vi "Teleop.vi"(10 "Match Info":T4={"Autonomous Elapsed Seconds"=0.0, "TeleOp Elapsed Seconds"=0.0, "Disabled Elapsed Seconds"=0.0, "Visited Autonomous"=FALSE, "Visited TeleOp"=FALSE, "Visited Disabled"=FALSE, "Autonomous Settings"={"Autonomous Style"=enum."Independent", "VI Refnum"=refnum}}, 11 "Call Context":T5) -> ()   [LabVIEW 2018]
doc: "This VI is called for each TeleOp packet received from the DS where the robot is not disabled. It is often used to read from the joysticks and update I/O or to update setpoints for timed control loops. It should complete and return within 20 milliseconds or it may miss DS packets."
uses:
  <vilib>/Rock Robotics/WPI/DriverStation/WPI_DriverStationDerivedRobotMode.ctl
  <vilib>/Rock Robotics/WPI/DriverStation/WPI_DriverStationMatch Info.ctl
  <vilib>/Rock Robotics/WPI/Solenoid/WPI_SolenoidValue.ctl
  <vilib>/Rock Robotics/WPI/ThirdParty/Phoenix-LabVIEW/Motor Controller/Controls/CTRE_Phoenix_MotorControl_ControlMode.ctl
  <vilib>/Rock Robotics/WPI/Switch/WPI_SwitchDevRef.ctl
  <vilib>/Rock Robotics/SystemInterfaces/DIO/FPGA_DIOChannel.ctl
  <vilib>/Rock Robotics/SystemInterfaces/Counter/FPGA_CounterCtrSystemIndex.ctl
  <vilib>/Rock Robotics/WPI/Utilities/WPI_GetSetVariantRefNum.vi
  <vilib>/Rock Robotics/WPI/Joystick/WPI_JoystickArcadeMapping.vi
  <vilib>/Rock Robotics/Network Tables/NT Write Boolean Array.vi
  <vilib>/Rock Robotics/Network Tables/NT Write Numeric Array.vi
  <vilib>/Rock Robotics/WPI/Solenoid/WPI_SolenoidSetEnum.vi
  <vilib>/Rock Robotics/WPI/ThirdParty/Phoenix-LabVIEW/Motor Controller/Get/CTRE_Phoenix_MotorController_GetSelectedSensorData.vi
  <vilib>/Rock Robotics/Network Tables/NT Read Boolean.vi
  Toolbox/Simple Limit Switch/Limits(Switch+Encoder).vi
  Toolbox/Simple Limit Switch/Limits(DoubleEncoder).vi
  Toolbox/Simple Limit Switch/Limits(DoubleSwitch).vi
  <vilib>/Rock Robotics/Network Tables/NT Read Number.vi
panel:
  in  "Reset Elevator Horse":bool
  out "OuterStageSwitch":bool
  out "Wrist Indicator":T1(ring)
  out "Elevator Intake":T2(ring)
  in  "Wrist":T1(ring)
  in  "Level":T2(ring)
  in  "Elevator Auto":bool
  in  "Elevator Output Range":cluster{"output high":dbl, "output low":dbl}={"output high"=0.25, "output low"=-0.25}
  in  "Elevator PID Gains":T3={"proportional gain (Kc)"=1.0, "integral time (Ti, min)"=0.01, "derivative time (Td, min)"=0.0}
  in  "Elevator Setpoints":dbl[](array[numeric])=[-1000.0, -100000.0, -250000.0, -250000.0, -270000.0, -480000.0]
  in  "Wrist Auto":bool
  in  "Wrist Output Range":cluster{"output high":dbl, "output low":dbl}={"output high"=0.25, "output low"=-0.25}
  in  "Wrist PID Gains":T3={"proportional gain (Kc)"=1.0, "integral time (Ti, min)"=0.01, "derivative time (Td, min)"=0.0}
  in  "Wrist Setpoints":dbl[](array[numeric])=[-34000.0, -34000.0, -34000.0, -34000.0, 120000.0, 50000.0, 38000.0, 0.0, -34000.0]
  in  "Level":i8
  in  "Into Home Limit Is Pos (Wrist)":bool
  out "Wrist Limit Switch":bool
  out "Elevator Limit Switch Top":bool
  in  "Into Home Limit Is Pos (Elevator)":bool=TRUE
  in  "Intake Encoder Limit":dbl=560000.0 format="%#_13g"
  in  "Intake Home Encoder Limit":dbl=-100000.0 format="%#_13g"
  in  "HorseDanger":i32=700
  in  "Horse Encoder Limit":dbl=180000.0 format="%#_13g"
  in  "Into Home Limit Is Pos (Horse)":bool
  out "Elevator Limit Switch":bool
  out "Elevator Encoder":i32
  in  "Reset Elevator Encoder":bool
  out "Horse Encoder":i32
  in  "Reset Wrist Encoder":bool
  out "Intake Wrist Encoder":i32
  # "UNKNOWN"
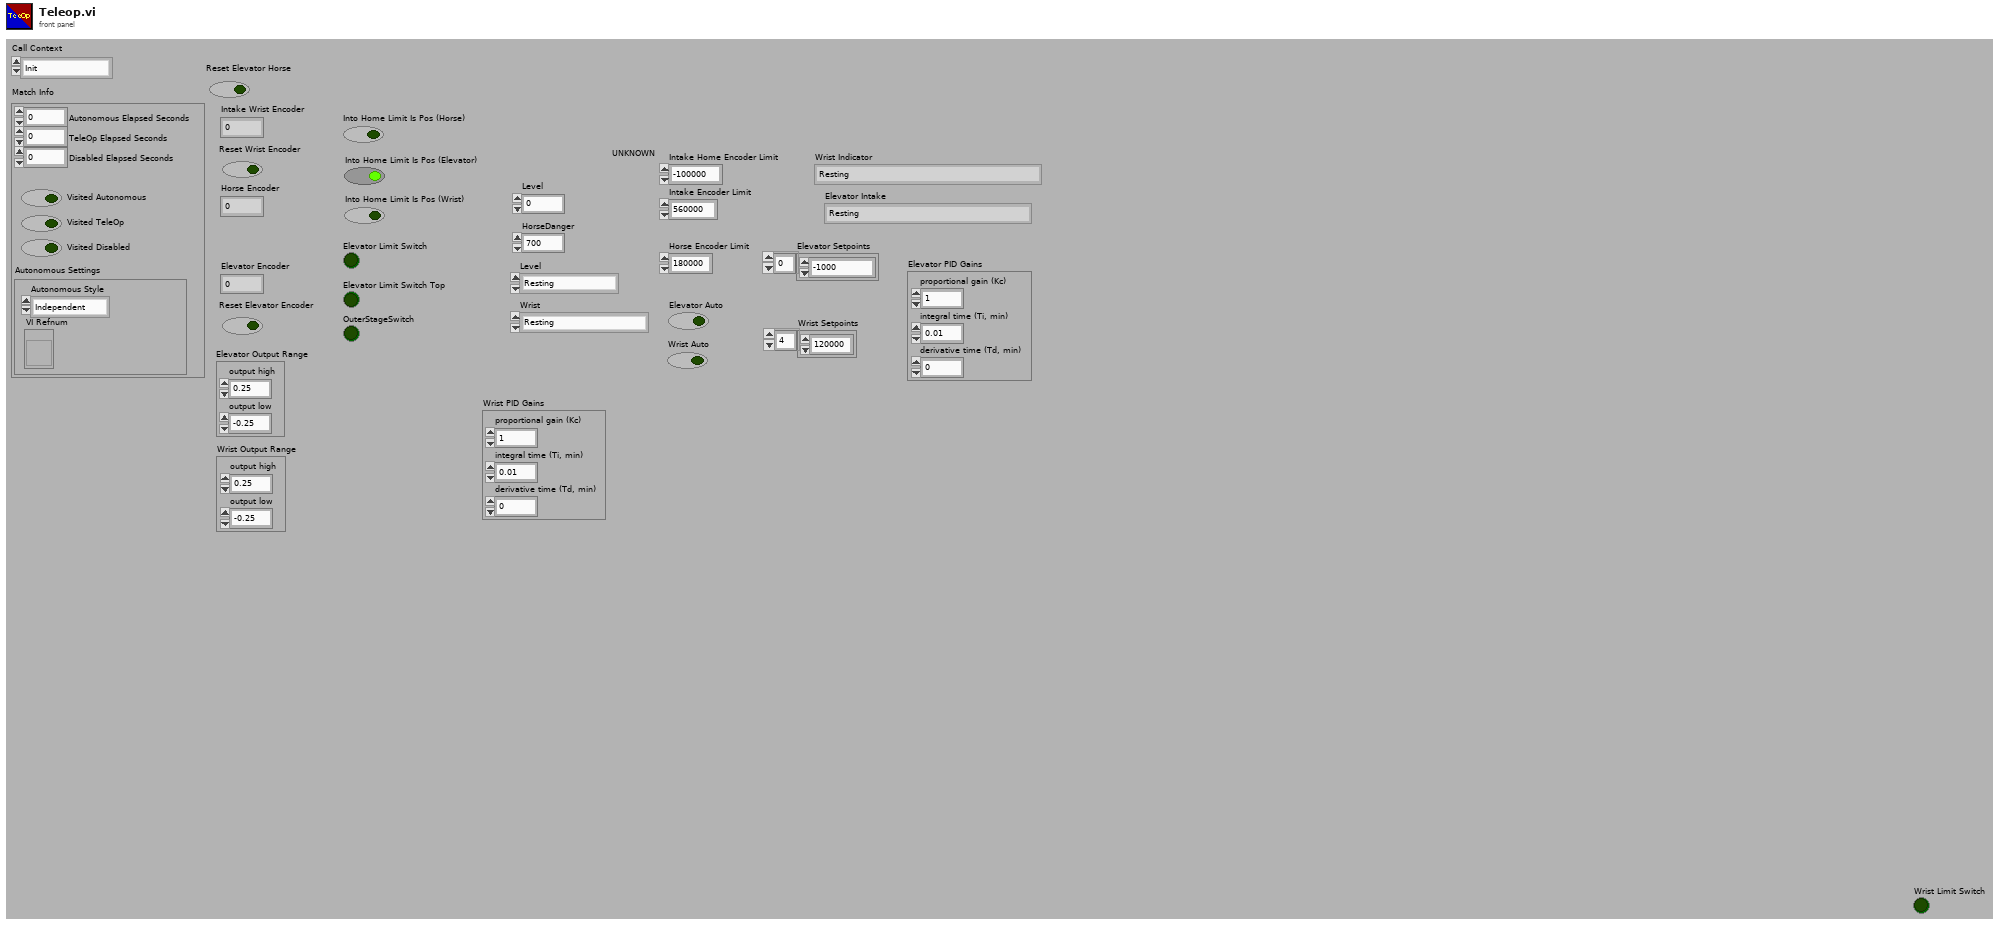
[diagram p1: front panel]
types:
  T1 = enum16{"Resting", "Hatch Ground Intake", "Hatch Place Low/Mid/CargoShip", "Hatch Place High", "Cargo Ground Intake", "Cargo Place Low/Mid", "Cargo Place High", "CargoShip Place Front", "CargoShip Place Back"}
  T2 = enum16{"Resting", "CargoShip Front", "CargoShip Back", "Cargo Mid", "Hatch Mid", "All High"}
  T3 = cluster{"proportional gain (Kc)":dbl, "integral time (Ti, min)":dbl, "derivative time (Td, min)":dbl}
  T4 = typedef "WPI_DriverStationMatch Info.ctl" = cluster{"Autonomous Elapsed Seconds":dbl, "TeleOp Elapsed Seconds":dbl, "Disabled Elapsed Seconds":dbl, "Visited Autonomous":bool, "Visited TeleOp":bool, "Visited Disabled":bool, "Autonomous Settings":cluster{"Autonomous Style":enum16{"Iterative", "Independent"}, "VI Refnum":refnum<vi>}}
  T5 = typedef "WPI_DriverStationDerivedRobotMode.ctl" = enum16{"Init", "Execute", "Stop"}
  T6 = typedef "WPI_SwitchDevRef.ctl" = cluster{"DevStatus":errorcluster, "DIO Channel":T7, "CntIndex":T8, "Normally Closed":bool}
  T7 = typedef "FPGA_DIOChannel.ctl" = enum8{"DIO 0", "DIO 1", "DIO 2", "DIO 3", "DIO 4", "DIO 5", "DIO 6", "DIO 7", "DIO 8", "DIO 9", "DIO MXP 0", "DIO MXP 1", "DIO MXP 2", "DIO MXP 3", "DIO MXP 4", "DIO MXP 5", "DIO MXP 6", "DIO MXP 7", "DIO MXP 8", "DIO MXP 9", "DIO MXP 10", "DIO MXP 11", "DIO MXP 12", "DIO MXP 13", "DIO MXP 14", "DIO MXP 15", "SPI Port CS1", "SPI Port CS2", "SPI Port CS3", "SPI Port MISO", "SPI Port MOSI", "Invalid"}
  T8 = typedef "FPGA_CounterCtrSystemIndex.ctl" = enum8{"Ctr 0", "Ctr 1", "Ctr 2", "Ctr 3", "Ctr 4", "Ctr 5", "Ctr 6", "Ctr 7", "Invalid"}
  T9 = cluster{"Increment Setpoint Index":bool, "Decrement Setpoint Index":bool}
  T10 = typedef "CTRE_Phoenix_MotorControl_ControlMode.ctl" = u16
  T11 = typedef "WPI_SolenoidValue.ctl" = enum16{"Off", "On", "Forward", "Reverse"}
  T12 = cluster{"Intake Wheels Forwards":bool, "Elevator Shift":bool, "Intake Wheels Backwards":bool, "Drivetrain Shift":bool, "Elevator Outer Forwards":bool, "Elevator Outer Backwards":bool, "Horse Drive Climber":bool, "Horse Drive Pistons":bool, "Horse Drive Up":bool, "Horse Drive Down":bool}
  T13 = typedef "WPI_JoystickDevRef.ctl" = cluster{"Device":T14}
  T14 = typedef "WPI_JoystickDeviceEnum.ctl" = enum16{"USB 0", "USB 1", "USB 2", "USB 3", "USB 4", "USB 5"}
  T15 = typedef "WPI_MotorControlDeviceRef.ctl" = cluster{"DeviceStatus":errorcluster, "Type":T16, "PWM":cluster{"PWM Channel":T17, "DeadBand":T18}, "CAN":cluster{"Device Number":u8, "SetOutput VI Ref":variant, "GetOutput VI Ref":variant, "Enable VI Ref":variant, "Disable VI Ref":variant, "Data":variant}, "Invert":bool, "DIO PWM":cluster{"PWM \"Enable\" Channel":T17, "DIOChannel":T7, "PWM Rate":dbl}}
  T16 = typedef "WPI_MotorControlType.ctl" = enum16{"PWM", "CAN", "DIO PWM"}
  T17 = typedef "FPGA_DIOPWMChannel.ctl" = enum8{"PWM 0", "PWM 1", "PWM 2", "PWM 3", "PWM 4", "PWM 5", "PWM 6", "PWM 7", "PWM 8", "PWM 9", "PWM MXP 0", "PWM MXP 1", "PWM MXP 2", "PWM MXP 3", "PWM MXP 4", "PWM MXP 5", "PWM MXP 6", "PWM MXP 7", "PWM MXP 8", "PWM MXP 9", "Invalid"}
  T18 = typedef "WPI_PWMDeadband.ctl" = cluster{"Name":string, "maxPositivePwm":i32, "minPositivePwm":i32, "centerPwm":i32, "maxNegativePwm":i32, "minNegativePwm":i32, "angularRange":u16}
  T19 = cluster{"Elevator Setpoints":dbl[], "Wrist Setpoints":dbl[], "Horse Drive Setpoints":dbl[], "Wrist Gains":cluster{"proportional gain (Kc)":dbl, "integral time (Ti, min)":dbl, "derivative time (Td, min)":dbl}, "Wrist Power Limits":cluster{"output high":dbl, "output low":dbl}, "Horse Gains":cluster{"proportional gain (Kc)":dbl, "integral time (Ti, min)":dbl, "derivative time (Td, min)":dbl}, "Horse Power Limits":cluster{"output high":dbl, "output low":dbl}, "Elevator Gains":cluster{"proportional gain (Kc)":dbl, "integral time (Ti, min)":dbl, "derivative time (Td, min)":dbl}, "Elevator Power Limits":cluster{"output high":dbl, "output low":dbl}}
  T20 = enum16{"Resting", "CargoShip Front", "CargoShip Back", "Cargo Mid", "Hatch Mid", "All High", "Cargo Intake"}
  T21 = typedef "WPI_SolenoidDevRef.ctl" = cluster{"DevStatus":errorcluster, "Pneumatics Control Module":u8, "Forward Solenoid Channel":T22, "Reverse Solenoid Channel":T22}
  T22 = typedef "WPI_SolenoidChannel.ctl" = enum8{"Solenoid 0", "Solenoid 1", "Solenoid 2", "Solenoid 3", "Solenoid 4", "Solenoid 5", "Solenoid 6", "Solenoid 7", "Invalid"}
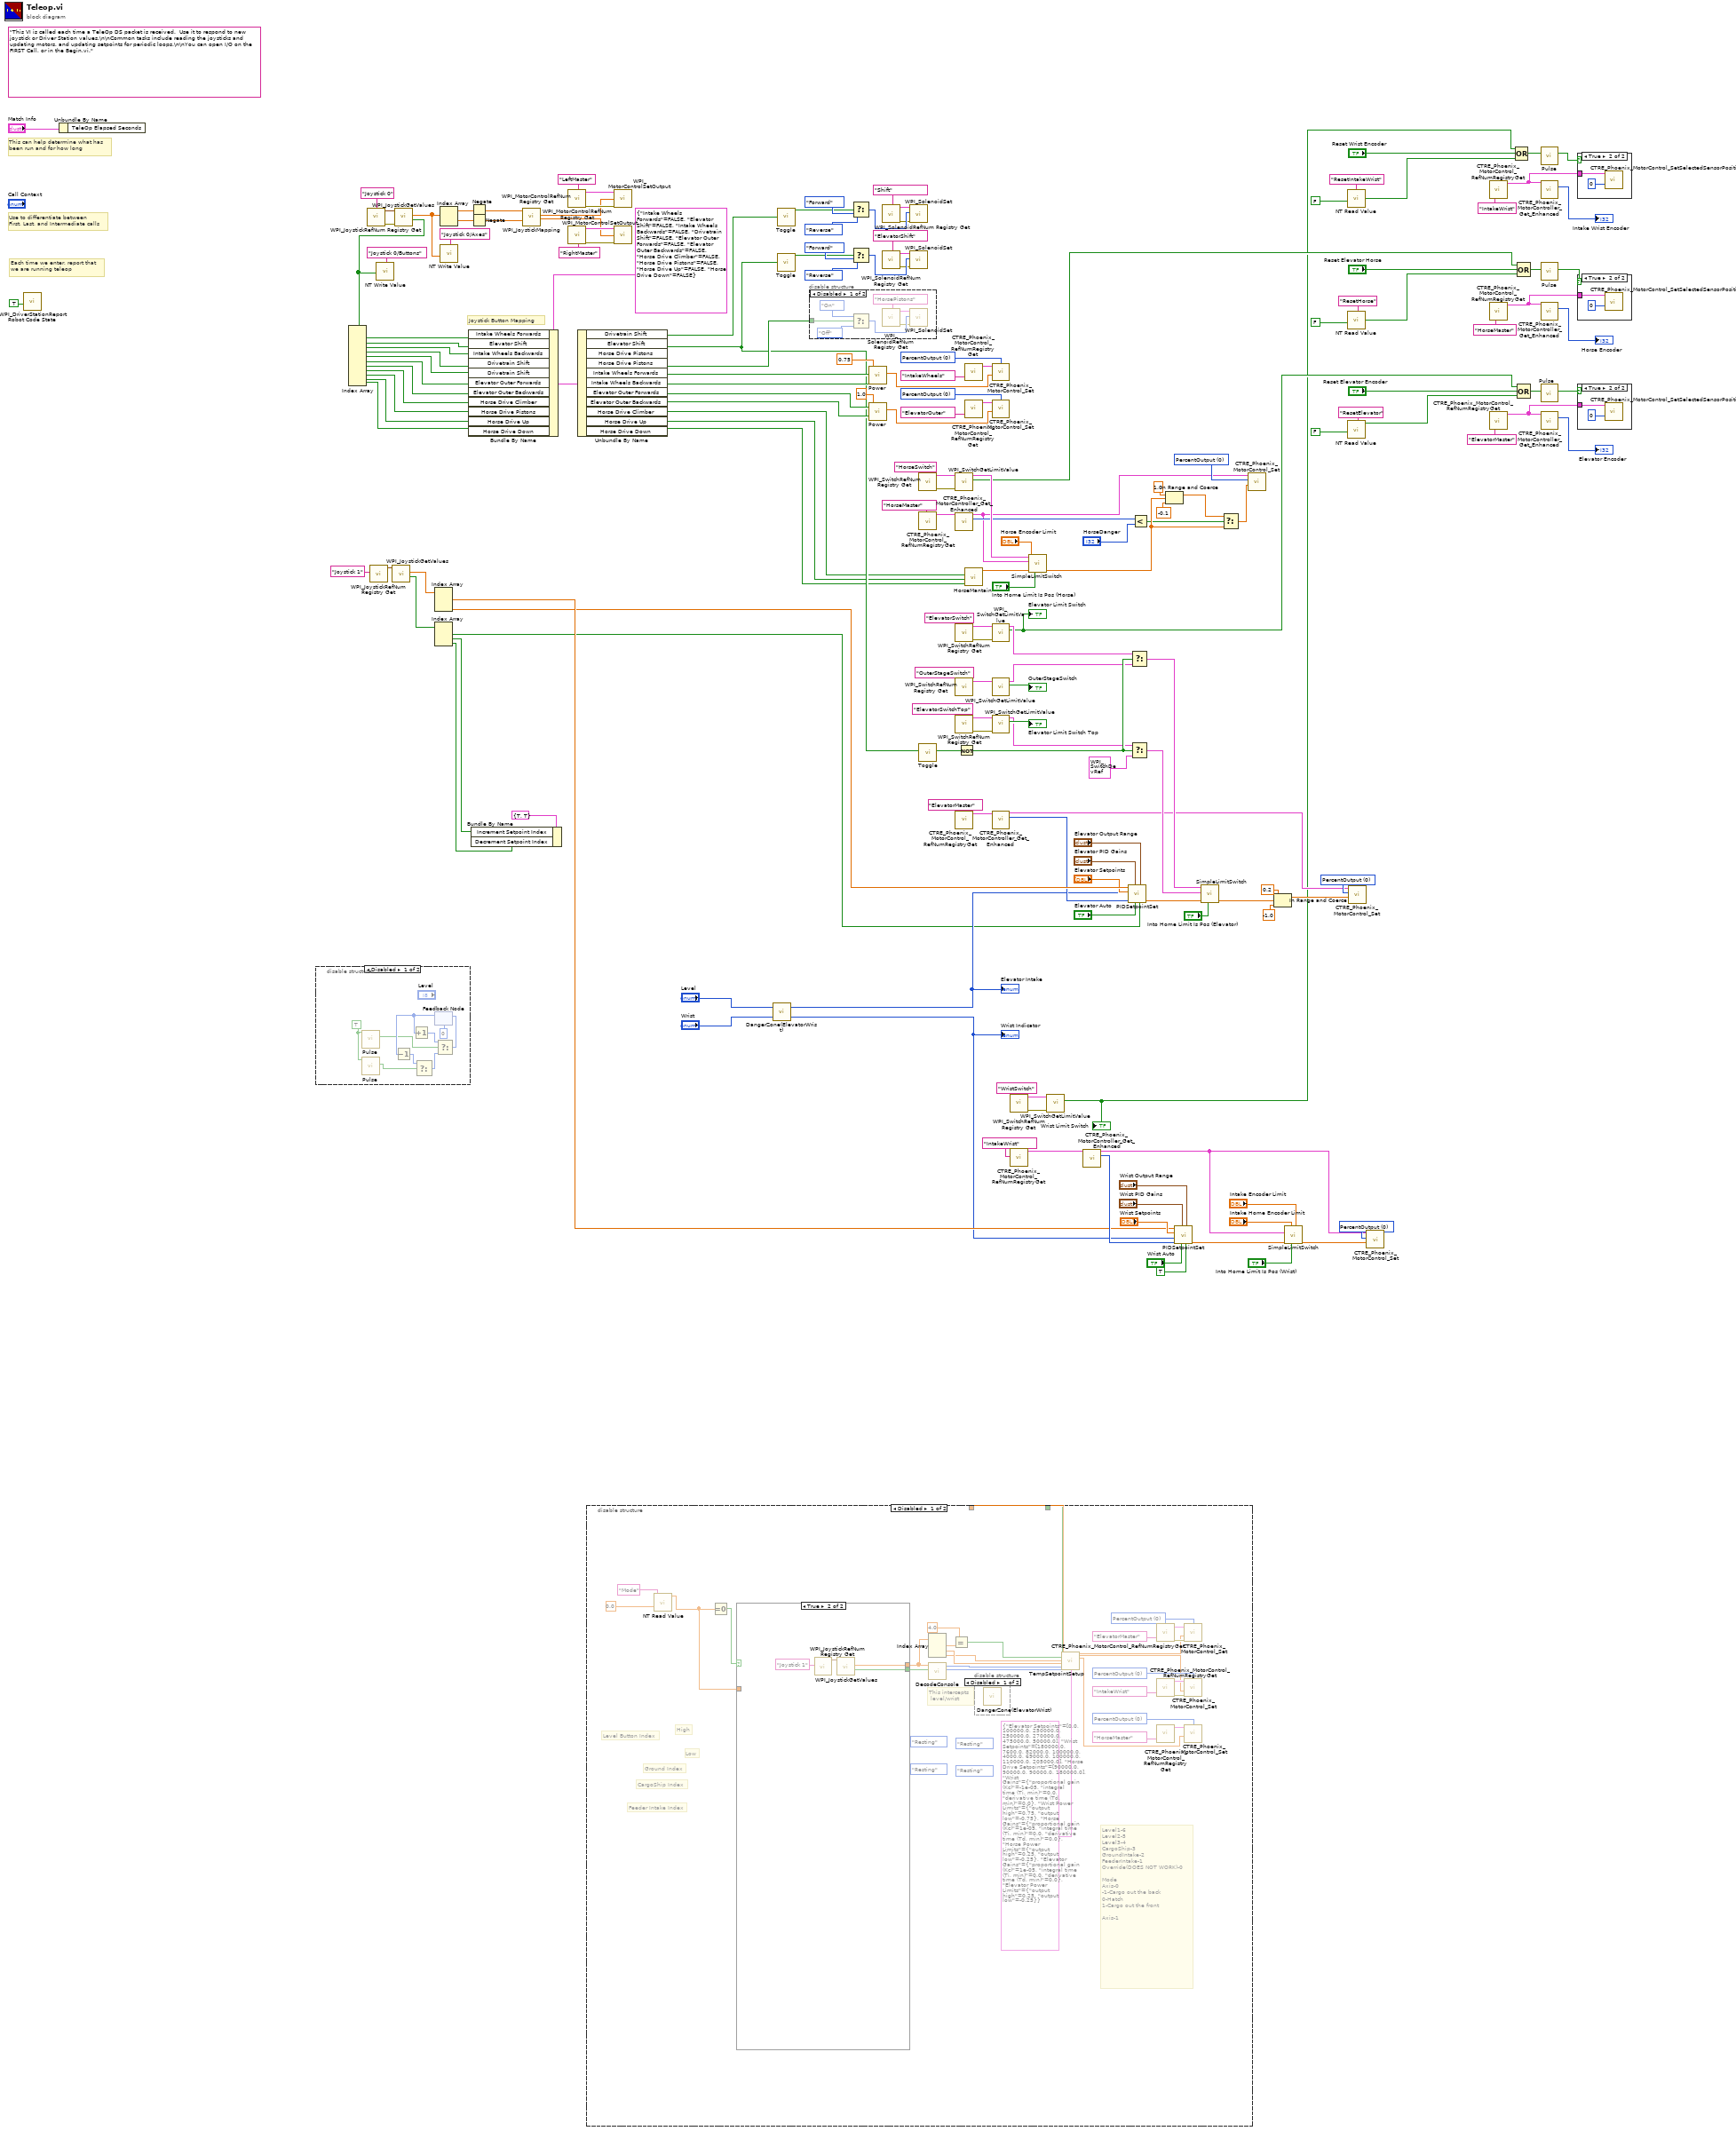
[diagram p0: block diagram]
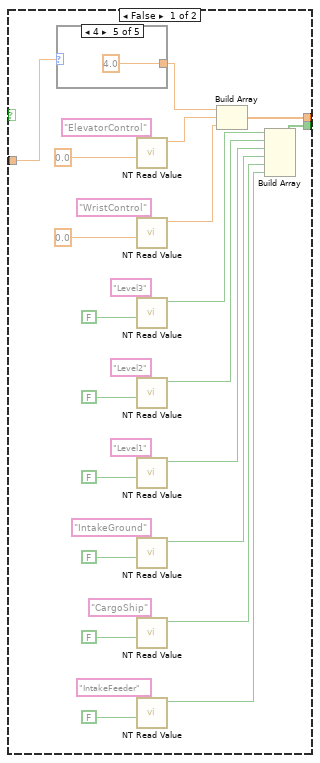
[diagram p8: hidden frame]
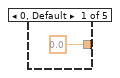
[diagram p9: hidden frame]
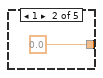
[diagram p10: hidden frame]
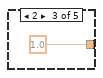
[diagram p11: hidden frame]
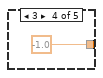
[diagram p12: hidden frame]
diagram:
  w73 = T10 0 items=["PercentOutput"=0, "Position"=1, "Velocity"=2, "Current"=3, "Follower"=5, "MotionProfile"=6, "MotionMagic"=7, "MotionProfileArc"=10, "Disabled"=15] ("Control Mode")
  w10 = T10 0 items=["PercentOutput"=0, "Position"=1, "Velocity"=2, "Current"=3, "Follower"=5, "MotionProfile"=6, "MotionMagic"=7, "MotionProfileArc"=10, "Disabled"=15] ("Control Mode")
  w90 = T10 0 items=["PercentOutput"=0, "Position"=1, "Velocity"=2, "Current"=3, "Follower"=5, "MotionProfile"=6, "MotionMagic"=7, "MotionProfileArc"=10, "Disabled"=15] ("Control Mode")
  w100 = T10 0 items=["PercentOutput"=0, "Position"=1, "Velocity"=2, "Current"=3, "Follower"=5, "MotionProfile"=6, "MotionMagic"=7, "MotionProfileArc"=10, "Disabled"=15] ("Control Mode")
  w103 = T10 0 items=["PercentOutput"=0, "Position"=1, "Velocity"=2, "Current"=3, "Follower"=5, "MotionProfile"=6, "MotionMagic"=7, "MotionProfileArc"=10, "Disabled"=15] ("Control Mode")
  (unwired) "This VI is called each time a TeleOp DS packet is received.  Use it to respond to new joystick or Driver Station values.\n\nCommon tasks include reading the joysticks and updating motors, and updating setpoints for periodic loops.\n\nYou can open I/O on the FIRST Call, or in the Begin.vi."
  # "Joystick Button Mapping"
  # "Each time we enter, report that\nwe are running teleop"
  # "Use to differentiate between\nFirst, Last, and Intermediate calls"
  # "This can help determine what has\nbeen run and for how long"
  n1 = call <vilib>:"WPI_DriverStationReport Robot Code State.vi"("TeleOp"=TRUE ("Autonomous")) -> ()  [unwired: 10 in, 1 out]
  n2 = Unbundle By Name("Match Info") -> ()  [unwired: 1 out]
  n3 = disable-structure shown="Disabled" {
    frame Disabled {
      w182 = TRUE ("Rising Edge?")
      n4 = call "Pulse.vi"("Rising Edge?"=w182) -> ("Output"=w184:bool)  [unwired: 10 in]
      n5 = call "Pulse.vi"("Rising Edge?"=w182) -> ("Output"=w183:bool)  [unwired: 10 in]
      n6 = feedback #1(i8 0) -> (w186:i8)
      n7 = Decrement(x=w186) -> (x-1=w188:i8)
      n8 = Increment(x=w186) -> (x+1=w190:i8)
      n9 = Select(t=w188, s=w183) -> (s? t:f=w189:i8)  [unwired: 1 in]
      n10 = Select(t=w190, s=w184, f=w189) -> (s? t:f=w187:i8)
      n11 = feedback-in #1(w187) -> ()
    }
    frame Enabled {
    }
  }
  n12 = call <vilib>:"WPI_JoystickRefNum Registry Get.vi"("refnum name"="Joystick 0") -> ("error out"=w138:errorcluster, "JoystickDevRef"=w179:T13)  [unwired: 1 in, 8 out]
  n13 = call <vilib>:"WPI_JoystickRefNum Registry Get.vi"("refnum name"="Joystick 1") -> ("JoystickDevRef"=w82:T13)  [unwired: 9 in, 1 out]
  n14 = call <vilib>:"WPI_JoystickGetValues.vi"("JoystickDevRef"=w82) -> ("Buttons"=w55:bool[], "Axes"=w81:dbl[])  [unwired: 6 in, 3 out]
  n15 = call <vilib>:"WPI_JoystickGetValues.vi"("error in (no error)"=w138, "JoystickDevRef"=w179) -> ("Buttons"=w135:bool[], "Axes"=w175:dbl[])  [unwired: 5 in, 3 out]
  n16 = Index Array(array=w135) -> (element #1=w163:bool, element #2=w173:bool, element #3=w172:bool, element #4=w171:bool, element #5=w170:bool, element #6=w169:bool, element #7=w168:bool, element #8=w167:bool, element #9=w166:bool, element #10=w165:bool, element #11=w164:bool)  [unwired: 11 in]
  n17 = call-poly <vilib>:"NT Write Value.vi"("Boolean Array"=w135, "Name"="Joystick 0/Buttons") -> ()  [unwired: 9 in, 1 out]
  n18 = Index Array(array=w81) -> (element #1=w61:dbl, element #3=w50:dbl)  [unwired: 3 in, 1 out]
  n19 = Index Array(array=w55) -> (element #1=w41:bool, element #2=w53:bool, element #3=w52:bool)  [unwired: 3 in]
  n20 = Index Array(array=w175) -> (element #1=w108:dbl, element #2=w134:dbl)  [unwired: 2 in]
  n21 = call-poly <vilib>:"NT Write Value.vi"("Numeric Array"=w175, "Name"="Joystick 0/Axes") -> ()  [unwired: 9 in, 1 out]
  n22 = Bundle By Name(cluster=T12 {"Intake Wheels Forwards"=FALSE, "Elevator Shift"=FALSE, "Intake Wheels Backwards"=FALSE, "Drivetrain Shift"=FALSE, "Elevator Outer Forwards"=FALSE, "Elevator Outer Backwards"=FALSE, "Horse Drive Climber"=FALSE, "Horse Drive Pistons"=FALSE, "Horse Drive Up"=FALSE, "Horse Drive Down"=FALSE} ("input cluster"), "Intake Wheels Forwards"=w163, "Elevator Shift"=w173, "Intake Wheels Backwards"=w172, "Drivetrain Shift"=w171, "Drivetrain Shift"=w170, "Elevator Outer Forwards"=w169, "Elevator Outer Backwards"=w168, "Horse Drive Climber"=w167, "Horse Drive Pistons"=w166, "Horse Drive Up"=w165, "Horse Drive Down"=w164) -> (w162:T12)
  n23 = Negate(x=w108) -> (-x=w107:dbl)
  n24 = Negate(x=w134) -> (-x=w109:dbl)
  n25 = Bundle By Name(cluster=T9 {"Increment Setpoint Index"=TRUE, "Decrement Setpoint Index"=TRUE} ("input cluster"), "Increment Setpoint Index"=w53, "Decrement Setpoint Index"=w52) -> ()  [unwired: 1 out]
  n26 = call-poly <vilib>:"WPI_JoystickMapping.vi"("Y axis value"=w109, "X axis value"=w107) -> ("Right Motor Value"=w139:dbl, "Left Motor Value"=w140:dbl)  [unwired: 8 in]
  n27 = call <vilib>:"WPI_MotorControlRefNum Registry Get.vi"("refnum name"="LeftMaster") -> ("error out"=w145:errorcluster, "MotorControlDevRef"=w146:T15)  [unwired: 9 in]
  n28 = call <vilib>:"WPI_MotorControlRefNum Registry Get.vi"("refnum name"="RightMaster") -> ("error out"=w144:errorcluster, "MotorControlDevRef"=w143:T15)  [unwired: 9 in]
  n29 = Unbundle By Name(w162) -> ("Drivetrain Shift"=w133:bool, "Elevator Shift"=w35:bool, "Horse Drive Pistons"=w80:bool, "Intake Wheels Forwards"=w150:bool, "Intake Wheels Backwards"=w149:bool, "Elevator Outer Forwards"=w148:bool, "Elevator Outer Backwards"=w147:bool, "Horse Drive Climber"=w28:bool, "Horse Drive Up"=w30:bool, "Horse Drive Down"=w29:bool)  [unwired: 1 out]
  n30 = disable-structure shown="Disabled" {
    disable-tunnel: _ -> [w192 _]
    disable-tunnel: _ -> [w191 _]
    frame Disabled {
      w194 = T10 0 items=["PercentOutput"=0, "Position"=1, "Velocity"=2, "Current"=3, "Follower"=5, "MotionProfile"=6, "MotionMagic"=7, "MotionProfileArc"=10, "Disabled"=15] ("Control Mode")
      w201 = T10 0 items=["PercentOutput"=0, "Position"=1, "Velocity"=2, "Current"=3, "Follower"=5, "MotionProfile"=6, "MotionMagic"=7, "MotionProfileArc"=10, "Disabled"=15] ("Control Mode")
      w204 = T10 0 items=["PercentOutput"=0, "Position"=1, "Velocity"=2, "Current"=3, "Follower"=5, "MotionProfile"=6, "MotionMagic"=7, "MotionProfileArc"=10, "Disabled"=15] ("Control Mode")
      (unwired) T20."Resting" ("Elevator Level Select")
      (unwired) T20."Resting" ("Elevator Level Select")
      (unwired) T1."Resting" ("Wrist")
      (unwired) T1."Resting" ("Wrist")
      # "This intercepts\n level/wrist"
      # "Level1-6\nLevel2-5\nLevel3-4\nCargoShip-3\nGroundIntake-2\nFeederIntake-1\nOverride(DOES NOT WORK)-0\n\nMode\nAxis-0\n-1-Cargo out the back\n0-Hatch\n1-Cargo out the front\n\nAxis-1"
      # "CargoShip Index"
      # "Low"
      # "High"
      # "Feeder Intake Index"
      # "Ground Index"
      # "Level Button Index"
      n31 = call-poly <vilib>:"NT Read Value.vi"("Default Value"=0.0, "Name"="Mode") -> ("Numeric"=w216:dbl)  [unwired: 8 in, 1 out]
      n32 = Equal To 0?(x=w216) -> (x = 0?=w218:bool)
      n33 = case shown="True" w218 {
        tunnel: [w242 w255] -> w213
        tunnel: [w223 w254] -> w217
        tunnel: w216 -> [w222 _]
        frame False {
          n34 = case shown="4" w222 {
            tunnel: [0.0 0.0 1.0 -1.0 4.0] -> w221
            frame 0, Default {
            }
            frame 1 {
            }
            frame 2 {
            }
            frame 3 {
            }
            frame 4 {
            }
          }
          n35 = call-poly <vilib>:"NT Read Value.vi"("Default Value"=0.0, "Name"="ElevatorControl") -> ("Numeric"=w243:dbl)  [unwired: 8 in, 1 out]
          n36 = call-poly <vilib>:"NT Read Value.vi"("Default Value"=0.0, "Name"="WristControl") -> ("Numeric"=w244:dbl)  [unwired: 8 in, 1 out]
          n37 = call-poly <vilib>:"NT Read Value.vi"("Default Value"=FALSE, "Name"="Level3") -> ("Boolean"=w239:bool)  [unwired: 8 in, 1 out]
          n38 = call-poly <vilib>:"NT Read Value.vi"("Default Value"=FALSE, "Name"="Level2") -> ("Boolean"=w236:bool)  [unwired: 8 in, 1 out]
          n39 = call-poly <vilib>:"NT Read Value.vi"("Default Value"=FALSE, "Name"="Level1") -> ("Boolean"=w233:bool)  [unwired: 8 in, 1 out]
          n40 = call-poly <vilib>:"NT Read Value.vi"("Default Value"=FALSE, "Name"="IntakeGround") -> ("Boolean"=w230:bool)  [unwired: 8 in, 1 out]
          n41 = call-poly <vilib>:"NT Read Value.vi"("Default Value"=FALSE, "Name"="CargoShip") -> ("Boolean"=w227:bool)  [unwired: 8 in, 1 out]
          n42 = call-poly <vilib>:"NT Read Value.vi"("Default Value"=FALSE, "Name"="IntakeFeeder") -> ("Boolean"=w224:bool)  [unwired: 8 in, 1 out]
          n43 = Build Array(w221, w243, w244) -> (w242:dbl[])
          n44 = Build Array(w239, w236, w233, w230, w227, w224) -> (w223:bool[])
        }
        frame True {
          n45 = call <vilib>:"WPI_JoystickRefNum Registry Get.vi"("refnum name"="Joystick 1") -> ("JoystickDevRef"=w256:T13)  [unwired: 9 in, 1 out]
          n46 = call <vilib>:"WPI_JoystickGetValues.vi"("JoystickDevRef"=w256) -> ("Buttons"=w254:bool[], "Axes"=w255:dbl[])  [unwired: 6 in, 3 out]
        }
      }
      n47 = Index Array(array=w213) -> (element #1=w212:dbl, element #2=w209:dbl, element #3=w208:dbl)  [unwired: 3 in]
      n48 = call "DecodeConsole.vi"("Boolean Array"=w217, "Axis Array"=w213) -> ("Wrist"=w214:T1, "Elevator Level Select"=w215:T20)  [unwired: 8 in]
      n49 = Equal?(x=4.0, y=w212) -> (x = y?=w210:bool)
      n50 = disable-structure shown="Disabled" {
        frame Disabled {
          n51 = call "DangerZone(ElevatorWrist).vi"() -> ()  [unwired: 2 in, 2 out]
        }
        frame Enabled {
        }
      }
      n52 = call "TempSetpointSetup.vi"("Elevator Switch"=w191, "Enable Auto"=w210, "Elevator Manual Power"=w208, "Wrist Manual Power"=w209, "Horse Drive Manual Power"=w192, "Elevator Level Select"=w215, "Wrist"=w214, "Cluster"=T19 {"Elevator Setpoints"=[0.0, 100000.0, 250000.0, 250000.0, 270000.0, 475000.0, 50000.0], "Wrist Setpoints"=[180000.0, 7600.0, 82000.0, 100000.0, 4000.0, 69000.0, 100000.0, 110000.0, 205000.0], "Horse Drive Setpoints"=[90000.0, 90000.0, 90000.0, 180000.0], "Wrist Gains"={"proportional gain (Kc)"=-1e-05, "integral time (Ti, min)"=0.0, "derivative time (Td, min)"=0.0}, "Wrist Power Limits"={"output high"=0.75, "output low"=-0.75}, "Horse Gains"={"proportional gain (Kc)"=1e-05, "integral time (Ti, min)"=0.0, "derivative time (Td, min)"=0.0}, "Horse Power Limits"={"output high"=0.25, "output low"=-0.25}, "Elevator Gains"={"proportional gain (Kc)"=1e-05, "integral time (Ti, min)"=0.0, "derivative time (Td, min)"=0.0}, "Elevator Power Limits"={"output high"=0.25, "output low"=-0.25}}) -> ("Elevator Power Out"=w202:dbl, "Wrist Power Out"=w197:dbl, "Horse Drive Power Out"=w193:dbl)  [unwired: 17 in]
      n53 = call <vilib>:"CTRE_Phoenix_MotorControl_RefNumRegistryGet.vi"("refnum name"="ElevatorMaster") -> ("error out"=w203:errorcluster, "PhoenixMotorControlDevRef"=w205:T15)  [unwired: 9 in]
      n54 = call <vilib>:"CTRE_Phoenix_MotorControl_RefNumRegistryGet.vi"("refnum name"="IntakeWrist") -> ("error out"=w198:errorcluster, "PhoenixMotorControlDevRef"=w200:T15)  [unwired: 9 in]
      n55 = call <vilib>:"CTRE_Phoenix_MotorControl_RefNumRegistryGet.vi"("refnum name"="HorseMaster") -> ("PhoenixMotorControlDevRef"=w195:T15)  [unwired: 9 in, 1 out]
      n56 = call <vilib>:"CTRE_Phoenix_MotorControl_Set.vi"("error in (no error)"=w203, "Output"=w202, "Control Mode"=w204, "PhoenixMotorControlDevRef"=w205) -> ()  [unwired: 6 in, 2 out]
      n57 = call <vilib>:"CTRE_Phoenix_MotorControl_Set.vi"("error in (no error)"=w198, "Output"=w197, "Control Mode"=w201, "PhoenixMotorControlDevRef"=w200) -> ()  [unwired: 6 in, 2 out]
      n58 = call <vilib>:"CTRE_Phoenix_MotorControl_Set.vi"("Output"=w193, "Control Mode"=w194, "PhoenixMotorControlDevRef"=w195) -> ()  [unwired: 7 in, 2 out]
    }
    frame Enabled {
    }
  }
  n59 = call <vilib>:"WPI_MotorControlSetOutput.vi"("error in (no error)"=w145, "Output"=w140, "MotorControlDevRef"=w146) -> ()  [unwired: 6 in, 3 out]
  n60 = call <vilib>:"WPI_MotorControlSetOutput.vi"("error in (no error)"=w144, "Output"=w139, "MotorControlDevRef"=w143) -> ()  [unwired: 6 in, 3 out]
  n61 = call "DangerZone(ElevatorWrist).vi"("Wrist"="Wrist", "Level"="Level") -> ("Wrist"=w43:T1, "Level"=w44:T2)
  "Elevator Intake" <- w44
  "Wrist Indicator" <- w43
  n62 = call "Toggle.vi"("Input"=w133) -> ("Output"=w157:bool)  [unwired: 10 in]
  n63 = call "Toggle.vi"("Input"=w35) -> ("Output"=w94:bool)  [unwired: 10 in]
  n64 = disable-structure shown="Disabled" {
    disable-tunnel: w80 -> [w258 _]
    frame Disabled {
      n65 = Select(t=WPI_SolenoidValue."On" ("Value"), s=w258, f=WPI_SolenoidValue."Off" ("Value")) -> (s? t:f=w264:T11)
      n66 = call <vilib>:"WPI_SolenoidRefNum Registry Get.vi"("refnum name"="HorsePistons") -> ("error out"=w259:errorcluster, "SolenoidDevRef"=w261:T21)  [unwired: 9 in]
      n67 = call-poly <vilib>:"WPI_SolenoidSet.vi"("error in (no error)"=w259, "Value"=w264, "SolenoidDevRef"=w261) -> ()  [unwired: 7 in, 2 out]
    }
    frame Enabled {
    }
  }
  n68 = Select(t=WPI_SolenoidValue."Forward" ("Value"), s=w157, f=WPI_SolenoidValue."Reverse" ("Value")) -> (s? t:f=w156:T11)
  n69 = Select(t=WPI_SolenoidValue."Forward" ("Value"), s=w94, f=WPI_SolenoidValue."Reverse" ("Value")) -> (s? t:f=w155:T11)
  n70 = call "Power.vi"("Positive Power"=0.75 ("Power"), "Negative"=w149, "Positive"=w150) -> ("Output"=w102:dbl)  [unwired: 8 in]
  n71 = call "Power.vi"("Positive Power"=1.0 ("Power"), "Negative"=w147, "Positive"=w148) -> ("Output"=w101:dbl)  [unwired: 8 in]
  n72 = call <vilib>:"WPI_SolenoidRefNum Registry Get.vi"("refnum name"="Shift") -> ("error out"=w136:errorcluster, "SolenoidDevRef"=w160:T21)  [unwired: 9 in]
  n73 = call <vilib>:"WPI_SolenoidRefNum Registry Get.vi"("refnum name"="ElevatorShift") -> ("error out"=w137:errorcluster, "SolenoidDevRef"=w152:T21)  [unwired: 9 in]
  n74 = call-poly <vilib>:"WPI_SolenoidSet.vi"("error in (no error)"=w136, "Value"=w156, "SolenoidDevRef"=w160) -> ()  [unwired: 7 in, 2 out]
  n75 = call-poly <vilib>:"WPI_SolenoidSet.vi"("error in (no error)"=w137, "Value"=w155, "SolenoidDevRef"=w152) -> ()  [unwired: 7 in, 2 out]
  n76 = call <vilib>:"WPI_SwitchRefNum Registry Get.vi"("refnum name"="HorseSwitch") -> ("error out"=w96:errorcluster, "SwitchDevRef"=w89:T6)  [unwired: 9 in]
  n77 = call <vilib>:"CTRE_Phoenix_MotorControl_RefNumRegistryGet.vi"("refnum name"="HorseMaster") -> ("PhoenixMotorControlDevRef"=w16:T15)  [unwired: 9 in, 1 out]
  n78 = call "Toggle.vi"("Input"=w35) -> ("Output"=w24:bool)  [unwired: 10 in]
  n79 = call <vilib>:"WPI_SwitchGetLimitValue.vi"("error in (no error)"=w96, "SwitchDevRef"=w89) -> ("Switch Pressed"=w4:bool)  [unwired: 7 in, 2 out]
  n80 = call-poly <vilib>:"CTRE_Phoenix_MotorController_Get_Enhanced.vi"("PhoenixMotorControlDevRef"=w16) -> ("PhoenixMotorControlDevRef"=w1:T15, "Position (Raw Sensor Units)"=w86:i32)  [unwired: 11 in, 2 out]
  n81 = call <vilib>:"WPI_SwitchRefNum Registry Get.vi"("refnum name"="ElevatorSwitch") -> ("error out"=w92:errorcluster, "SwitchDevRef"=w34:T6)  [unwired: 9 in]
  n82 = call <vilib>:"WPI_SwitchRefNum Registry Get.vi"("refnum name"="OuterStageSwitch") -> ("SwitchDevRef"=w25:T6)  [unwired: 9 in, 1 out]
  n83 = call <vilib>:"WPI_SwitchRefNum Registry Get.vi"("refnum name"="ElevatorSwitchTop") -> ("error out"=w77:errorcluster, "SwitchDevRef"=w37:T6)  [unwired: 9 in]
  n84 = call <vilib>:"CTRE_Phoenix_MotorControl_RefNumRegistryGet.vi"("refnum name"="ElevatorMaster") -> ("PhoenixMotorControlDevRef"=w15:T15)  [unwired: 9 in, 1 out]
  n85 = Not(x=w24) -> (.not. x?=w23:bool)
  n86 = call <vilib>:"CTRE_Phoenix_MotorControl_RefNumRegistryGet.vi"("refnum name"="IntakeWheels") -> ("PhoenixMotorControlDevRef"=w104:T15)  [unwired: 9 in, 1 out]
  n87 = call <vilib>:"CTRE_Phoenix_MotorControl_RefNumRegistryGet.vi"("refnum name"="ElevatorOuter") -> ("PhoenixMotorControlDevRef"=w99:T15)  [unwired: 9 in, 1 out]
  n88 = call "HorseMantain.vi"("Negative"=w29, "Positive"=w30, "HorseToggle"=w28) -> ("Power"=w27:dbl)  [unwired: 8 in]
  n89 = call <vilib>:"CTRE_Phoenix_MotorControl_Set.vi"("Output"=w102, "Control Mode"=w103, "PhoenixMotorControlDevRef"=w104) -> ()  [unwired: 7 in, 2 out]
  n90 = call <vilib>:"CTRE_Phoenix_MotorControl_Set.vi"("Output"=w101, "Control Mode"=w100, "PhoenixMotorControlDevRef"=w99) -> ()  [unwired: 7 in, 2 out]
  n91 = call <vilib>:"WPI_SwitchGetLimitValue.vi"("error in (no error)"=w92, "SwitchDevRef"=w34) -> ("Switch Pressed"=w3:bool, "SwitchDevRef"=w14:T6)  [unwired: 7 in, 1 out]
  "Elevator Limit Switch" <- w3
  n92 = call <vilib>:"WPI_SwitchGetLimitValue.vi"("SwitchDevRef"=w25) -> ("Switch Pressed"=→"OuterStageSwitch":bool, "SwitchDevRef"=w13:T6)  [unwired: 8 in, 1 out]
  n93 = call <vilib>:"WPI_SwitchGetLimitValue.vi"("error in (no error)"=w77, "SwitchDevRef"=w37) -> ("Switch Pressed"=→"Elevator Limit Switch Top":bool, "SwitchDevRef"=w12:T6)  [unwired: 7 in, 1 out]
  n94 = call-poly <vilib>:"CTRE_Phoenix_MotorController_Get_Enhanced.vi"("PhoenixMotorControlDevRef"=w15) -> ("PhoenixMotorControlDevRef"=w11:T15, "Position (Raw Sensor Units)"=w49:i32)  [unwired: 11 in, 2 out]
  n95 = call <vilib>:"WPI_SwitchRefNum Registry Get.vi"("refnum name"="WristSwitch") -> ("error out"=w67:errorcluster, "SwitchDevRef"=w66:T6)  [unwired: 9 in]
  n96 = call <vilib>:"CTRE_Phoenix_MotorControl_RefNumRegistryGet.vi"("refnum name"="IntakeWrist") -> ("PhoenixMotorControlDevRef"=w57:T15)  [unwired: 9 in, 1 out]
  n97 = call-poly "SimpleLimitSwitch.vi"("Into Home Limit Is Pos (Motor)"="Into Home Limit Is Pos (Horse)", "Power In"=w27, "Encoder Limit"="Horse Encoder Limit", "Motor Ref"=w1, "Limit Switch Ref"=w89) -> ("Power Out"=w19:dbl)  [unwired: 6 in]
  n98 = call <vilib>:"WPI_SwitchGetLimitValue.vi"("error in (no error)"=w67, "SwitchDevRef"=w66) -> ("Switch Pressed"=w2:bool)  [unwired: 7 in, 2 out]
  "Wrist Limit Switch" <- w2
  n99 = call-poly <vilib>:"CTRE_Phoenix_MotorController_Get_Enhanced.vi"("PhoenixMotorControlDevRef"=w57) -> ("PhoenixMotorControlDevRef"=w9:T15, "Position (Raw Sensor Units)"=w63:i32)  [unwired: 11 in, 2 out]
  n100 = call "PIDSetpointSet.vi"("Update"=w41, "Output Range"="Elevator Output Range", "Auto"="Elevator Auto", "PID Gains"="Elevator PID Gains", "Encoder Position"=w49, "Level"=w44, "Setpoints"="Elevator Setpoints", "Manual Power"=w50) -> ("Power Out"=w48:dbl)  [unwired: 3 in]
  n101 = Select(t=w14, s=w23, f=w13) -> (s? t:f=w33:T6)
  n102 = Select(t=w12, s=w23, f=T6 {"DevStatus"={"status"=FALSE, "code"=0, "source"=""}, "DIO Channel"=enum."Invalid", "CntIndex"=enum."Invalid", "Normally Closed"=FALSE}) -> (s? t:f=w36:T6)
  n103 = Less?(x=w86, y="HorseDanger") -> (x < y?=w17:bool)
  n104 = In Range and Coerce(upper limit=1.0, x=w19, lower limit=-0.1) -> (coerced(x)=w20:dbl)  [unwired: 1 out]
  n105 = call "PIDSetpointSet.vi"("Update"=TRUE, "Output Range"="Wrist Output Range", "Auto"="Wrist Auto", "PID Gains"="Wrist PID Gains", "Encoder Position"=w63, "Level"=w43, "Setpoints"="Wrist Setpoints", "Manual Power"=w61) -> ("Power Out"=w60:dbl)  [unwired: 3 in]
  n106 = call-poly "SimpleLimitSwitch.vi"("Into Home Limit Is Pos"="Into Home Limit Is Pos (Elevator)", "Power In"=w48, "2nd Limit Switch Ref"=w36, "Home Limit Switch Ref"=w33) -> ("Power Out"=w71:dbl)  [unwired: 7 in]
  n107 = Select(t=w20, s=w17, f=w19) -> (s? t:f=w18:dbl)
  n108 = call <vilib>:"CTRE_Phoenix_MotorControl_Set.vi"("Output"=w18, "Control Mode"=w90, "PhoenixMotorControlDevRef"=w1) -> ()  [unwired: 7 in, 2 out]
  n109 = In Range and Coerce(upper limit=0.2, x=w71, lower limit=-1.0) -> (coerced(x)=w68:dbl)  [unwired: 1 out]
  n110 = call-poly "SimpleLimitSwitch.vi"("Encoder Limit"="Intake Encoder Limit", "Into Home Limit Is Pos (Motor)"="Into Home Limit Is Pos (Wrist)", "Home Encoder Limit"="Intake Home Encoder Limit", "Power In"=w60, "Motor Ref"=w9) -> ("Power Out"=w65:dbl)  [unwired: 6 in]
  n111 = call-poly <vilib>:"NT Read Value.vi"("Default Value"=FALSE, "Name"="ResetIntakeWrist") -> ("Boolean"=w118:bool)  [unwired: 8 in, 1 out]
  n112 = call-poly <vilib>:"NT Read Value.vi"("Default Value"=FALSE, "Name"="ResetHorse") -> ("Boolean"=w114:bool)  [unwired: 8 in, 1 out]
  n113 = call-poly <vilib>:"NT Read Value.vi"("Default Value"=FALSE, "Name"="ResetElevator") -> ("Boolean"=w8:bool)  [unwired: 8 in, 1 out]
  n114 = call <vilib>:"CTRE_Phoenix_MotorControl_Set.vi"("Output"=w68, "Control Mode"=w73, "PhoenixMotorControlDevRef"=w11) -> ()  [unwired: 7 in, 2 out]
  n115 = call <vilib>:"CTRE_Phoenix_MotorControl_Set.vi"("Output"=w65, "Control Mode"=w10, "PhoenixMotorControlDevRef"=w9) -> ()  [unwired: 7 in, 2 out]
  n116 = call <vilib>:"CTRE_Phoenix_MotorControl_RefNumRegistryGet.vi"("refnum name"="IntakeWrist") -> ("PhoenixMotorControlDevRef"=w130:T15)  [unwired: 9 in, 1 out]
  n117 = call <vilib>:"CTRE_Phoenix_MotorControl_RefNumRegistryGet.vi"("refnum name"="HorseMaster") -> ("PhoenixMotorControlDevRef"=w127:T15)  [unwired: 9 in, 1 out]
  n118 = call <vilib>:"CTRE_Phoenix_MotorControl_RefNumRegistryGet.vi"("refnum name"="ElevatorMaster") -> ("PhoenixMotorControlDevRef"=w122:T15)  [unwired: 9 in, 1 out]
  n119 = Compound Arithmetic op=OR(w2, "Reset Wrist Encoder", w118) -> (w120:bool)
  n120 = Compound Arithmetic op=OR(w4, "Reset Elevator Horse", w114) -> (w116:bool)
  n121 = Compound Arithmetic op=OR(w3, "Reset Elevator Encoder", w8) -> (w5:bool)
  n122 = call "Pulse.vi"("Input"=w120) -> ("Output"=w129:bool)  [unwired: 10 in]
  n123 = call-poly <vilib>:"CTRE_Phoenix_MotorController_Get_Enhanced.vi"("PhoenixMotorControlDevRef"=w130) -> ("Position (Raw Sensor Units)"=→"Intake Wrist Encoder":i32)  [unwired: 11 in, 3 out]
  n124 = call "Pulse.vi"("Input"=w116) -> ("Output"=w128:bool)  [unwired: 10 in]
  n125 = call-poly <vilib>:"CTRE_Phoenix_MotorController_Get_Enhanced.vi"("PhoenixMotorControlDevRef"=w127) -> ("Position (Raw Sensor Units)"=→"Horse Encoder":i32)  [unwired: 11 in, 3 out]
  n126 = call "Pulse.vi"("Input"=w5) -> ("Output"=w121:bool)  [unwired: 10 in]
  n127 = call-poly <vilib>:"CTRE_Phoenix_MotorController_Get_Enhanced.vi"("PhoenixMotorControlDevRef"=w122) -> ("Position (Raw Sensor Units)"=→"Elevator Encoder":i32)  [unwired: 11 in, 3 out]
  n128 = case shown="True" w129 {
    tunnel: w130 -> [_ w266]
    frame False {
    }
    frame True {
      n129 = call <vilib>:"CTRE_Phoenix_MotorControl_SetSelectedSensorPosition.vi"("New Sensor Position"=0, "PhoenixMotorControlDevRef"=w266) -> ()  [unwired: 8 in, 2 out]
    }
  }
  n130 = case shown="True" w128 {
    tunnel: w127 -> [_ w268]
    frame False {
    }
    frame True {
      n131 = call <vilib>:"CTRE_Phoenix_MotorControl_SetSelectedSensorPosition.vi"("New Sensor Position"=0, "PhoenixMotorControlDevRef"=w268) -> ()  [unwired: 8 in, 2 out]
    }
  }
  n132 = case shown="True" w121 {
    tunnel: w122 -> [_ w270]
    frame False {
    }
    frame True {
      n133 = call <vilib>:"CTRE_Phoenix_MotorControl_SetSelectedSensorPosition.vi"("New Sensor Position"=0, "PhoenixMotorControlDevRef"=w270) -> ()  [unwired: 8 in, 2 out]
    }
  }
